vi "Backlight Value.vi"(3 "Backlight":bool) -> (1 "BacklightVal":u8)   [LabVIEW 2020, in "CTI-Peripheral.lvlib" / "PCF8574 I2C LCD.lvclass"]
uses:
  PCF8574 I2C LCD.lvclass
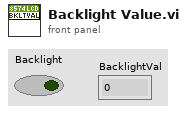
[diagram p1: front panel]
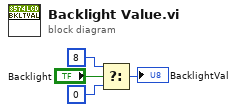
[diagram p0: block diagram]
diagram:
  n1 = Select(t=u8 8 ("BacklightVal"), s="Backlight", f=u8 0 ("BacklightVal")) -> (s? t:f=→"BacklightVal":u8)
